vi "Read Name Stuff.vi"(11 "Name Specs in":refnum<class "Name Specs.lvclass">) -> (2 "Name Stuff":T1)   [LabVIEW 2025, in "_Shared.lvlib" / "Name Specs.lvclass"]
uses:
  Name Specs.lvclass
  Name Stuff.ctl
  Type.ctl
  Name Specs.lvclass/Name Specs.ctl
  _Shared.lvlib
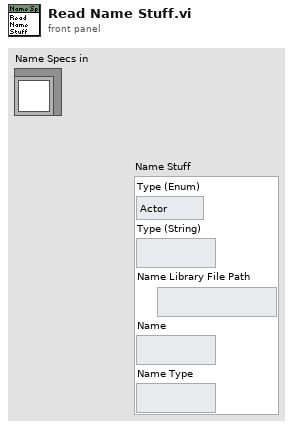
[diagram p1: front panel]
types:
  T1 = typedef "_Shared.lvlib/Name Stuff.ctl" = cluster{"Type (Enum)":T2, "Type (String)":string, "Name Library File Path":path, "Name":string, "Name Type":string}
  T2 = typedef "_Shared.lvlib/Type.ctl" = enum16{"Actor", "Msg"}
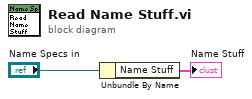
[diagram p0: block diagram]
diagram:
  n1 = Unbundle By Name("Name Specs in") -> ("Name Stuff"=→"Name Stuff":T1)
